vi "Configure Modulation (Frequency).vi"(0 "VISA resource name":refnum<visa-resource-name>, 1 "Modulation Frequency (100.00 Hz)":dbl=100.0, 2 "Peak Deviation (100.00 Hz)":dbl=100.0, 5 "Enable Frequency Modulation (T: Enable)":bool=TRUE, 7 "FM Source (0: Internal)":u16(ring) items=["Internal", "External"], 9 "Modulation Waveform (0: Sine)":i32(ring) items=["Sine", "Square", "Ramp", "Negative Ramp", "Triangle", "Noise", "Arbitrary Waveform"], 11 "error in (no error)":errorcluster) -> (4 "VISA resource name out":refnum<visa-resource-name>, 15 "error out":errorcluster)   [LabVIEW 2010, in "Agilent 33XXX Series.lvlib"]
doc: "Configures and enables frequency modulation (FM). In FM, the frequency of the carrier is varied by the frequency of the modulating waveform. \n\nNote: The carrier waveform shape and parameters are set by the Configure Standard Waveform vi."
uses:
  <instrlib>/Agilent 33XXX Series/Agilent 33XXX Series.lvlib
panel:
  # "Internal FM Settings"
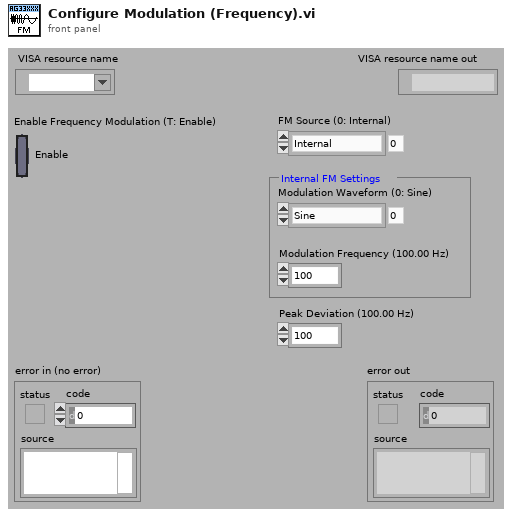
[diagram p1: front panel]
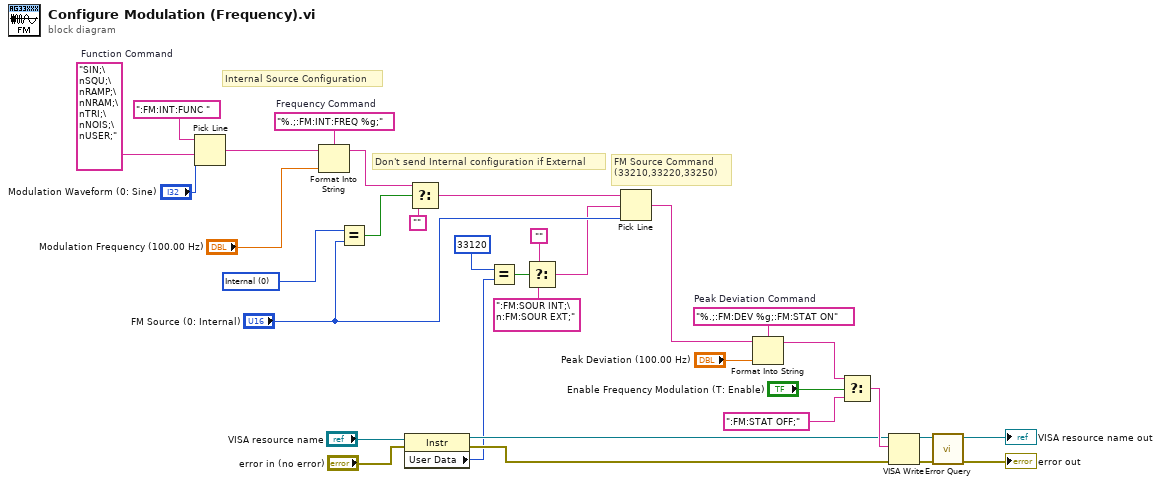
[diagram p0: block diagram]
diagram:
  w26 = "SIN;\nSQU;\nRAMP;\nNRAM;\nTRI;\nNOIS;\nUSER;"  # Function Command
  w27 = "%.;:FM:INT:FREQ %g;"  # Frequency Command
  w31 = "%.;:FM:DEV %g;:FM:STAT ON"  # Peak Deviation Command
  w21 = u16 0 items=["Internal", "External"] ("Source (0: Internal)")
  # "Internal Source Configuration"
  # "Don't send Internal configuration if External"
  # "FM Source Command\n(33210,33220,33250)"
  n1 = Pick Line(string ("")=":FM:INT:FUNC ", multi-line string=w26, line index="Modulation Waveform (0: Sine)") -> (output string=w22:string)
  n2 = Format Into String(format string=w27, initial string=w22, "Modulation Frequency (100.00 Hz)") -> (resulting string=w24:string)  [unwired: 1 in, 1 out]
  n3 = Equal?(x=w21, y="FM Source (0: Internal)") -> (x = y?=w13:bool)
  n4 = property class="Instr"(reference="VISA resource name", error in="error in (no error)") -> (reference out=w19:refnum<visa-resource-name>, error out=w18:errorcluster, "User Data"=w17:u32)
  n5 = Select(t=w24, s=w13, f="") -> (s? t:f=w11:string)
  n6 = Equal?(x=u32 33120, y=w17) -> (x = y?=w12:bool)
  n7 = Select(t="", s=w12, f=":FM:SOUR INT;\n:FM:SOUR EXT;" ("Source Command")) -> (s? t:f=w7:string)
  n8 = Pick Line(string ("")=w11, multi-line string=w7, line index="FM Source (0: Internal)") -> (output string=w10:string)
  n9 = Format Into String(format string=w31, initial string=w10, "Peak Deviation (100.00 Hz)") -> (resulting string=w9:string)  [unwired: 1 in, 1 out]
  n10 = Select(t=w9, s="Enable Frequency Modulation (T: Enable)", f=":FM:STAT OFF;") -> (s? t:f=w23:string)
  n11 = VISA Write(VISA resource name=w19, write buffer=w23, error in (no error)=w18) -> (VISA resource name out=w32:refnum<visa-resource-name>, error out=w33:errorcluster)  [unwired: 1 out]
  n12 = call <instrlib>:"Error Query.vi"("error in (no error)"=w33, "VISA resource name"=w32) -> ("error out"=→"error out":errorcluster, "VISA resource name out"=→"VISA resource name out":refnum<visa-resource-name>)  [unwired: 6 in, 2 out]
